vi "OAT Edge Detection.vi"   [LabVIEW 2017, in "SoundVib_TachProcess.lvlib"]
uses:
  <vilib>/addons/Sound and Vibration/Order Analysis/Tach Process/SoundVib_TachProcess.lvlib
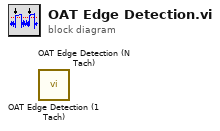
[diagram p0: block diagram]
diagram:
  n1 = call <vilib>:"OAT Edge Detection (1 Tach).vi"() -> ()  [unwired: 10 in, 2 out]
  n2 = call <vilib>:"OAT Edge Detection (N Tach).vi"() -> ()  [unwired: 10 in, 2 out]
